vi "temperature.vi"   [LabVIEW 2011]
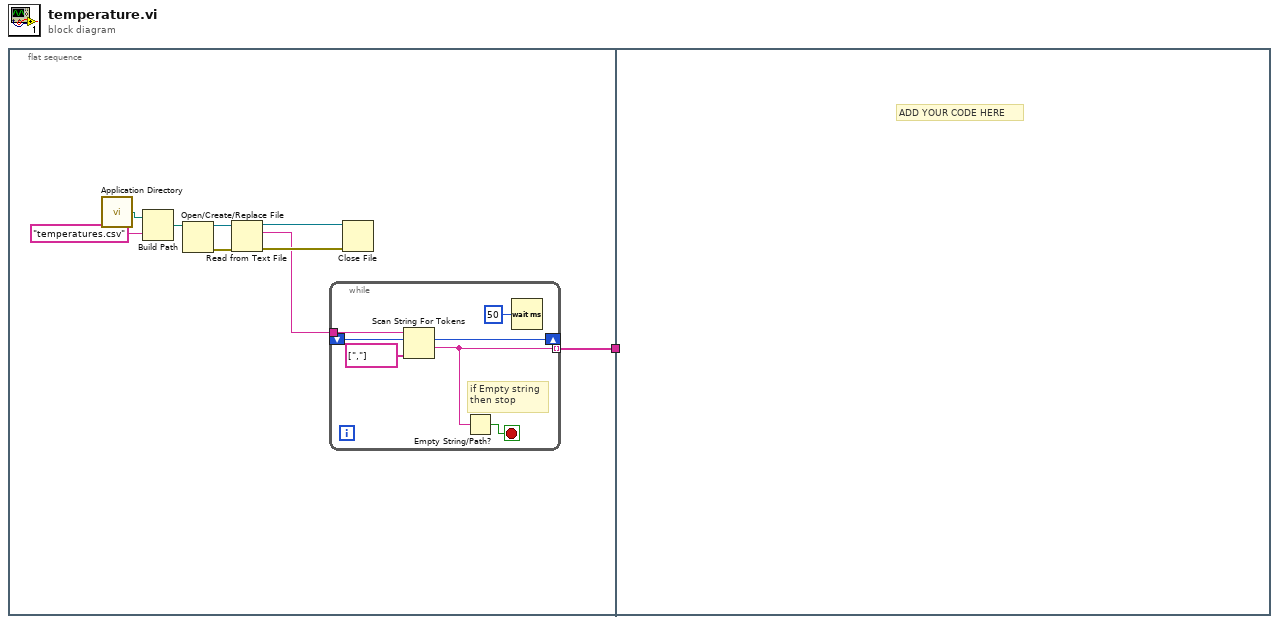
[diagram p0: block diagram]
diagram:
  n1 = flat-sequence {
    tunnel: [w5] -> w1
    tunnel: w1 -> [_]
    frame #0 {
      n2 = call <vilib>:"Application Directory.vi"() -> ("Application Directory"=w2:path)
      n3 = Build Path(base path=w2, name or relative path="temperatures.csv") -> (appended path=w4:path)
      n4 = Open/Create/Replace File(file path (use dialog)=w4) -> (refnum out=w10:refnum<file>, error out=w7:errorcluster)  [unwired: 5 in, 1 out]
      n5 = Read from Text File(file (use dialog)=w10, error in=w7) -> (refnum out=w9:refnum<file>, text=w6:string, error out=w8:errorcluster)  [unwired: 2 in, 1 out]
      n6 = while {
        tunnel: w6 -> [w17]
        tunnel: [w15] -> w5 mode=indexing
        shift-right: [w12] -> _
        shift-left: _ -> [w11]
        stop <- w16 stop-if-true
        # "if Empty string\nthen stop"
        n7 = Scan String For Tokens(6:string[] [","] ("delimiters (\\s,\\t,\\r,\\n)"), 8:w11, 9:w17) -> (1:w15:string, 2:w12:i32)  [unwired: 3 in, 2 out]
        n8 = Empty String/Path?(string/path=w15) -> (empty?=w16:bool)
        n9 = Wait (ms)(milliseconds to wait=u32 50) -> ()  [unwired: 1 out]
      }
      n10 = Close File(refnum=w9, error in=w8) -> ()  [unwired: 2 out]
    }
    frame #1 {
      # "ADD YOUR CODE HERE"
    }
  }
